vi "Local Bus Termination.vi"(8 "error in (no error)":errorcluster, 11 "BoardHandle":T1) -> (0 "error out":errorcluster, 2 "Local Bus Termination ON?":bool, 3 "BoardHandle out":T1)   [LabVIEW 2020, in "CAEN PSM.lvlib"]
doc: "This function returns bus termination status. (This is supported by NIM / DESKTOP HV family)."
uses:
  CAEN PSM.lvlib
  Private/BoardHandle.ctl
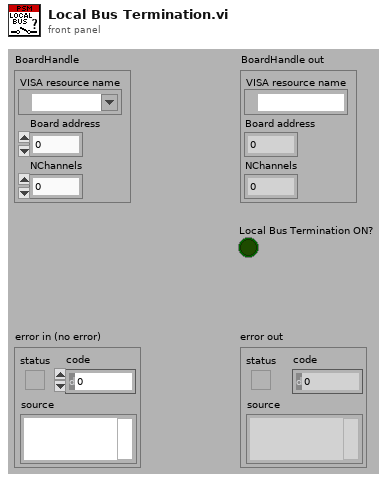
[diagram p1: front panel]
types:
  T1 = typedef "CAEN PSM.lvlib/BoardHandle.ctl" = cluster{"VISA resource name":refnum<visa-resource-name>, "Board address":i8, "NChannels":u8}
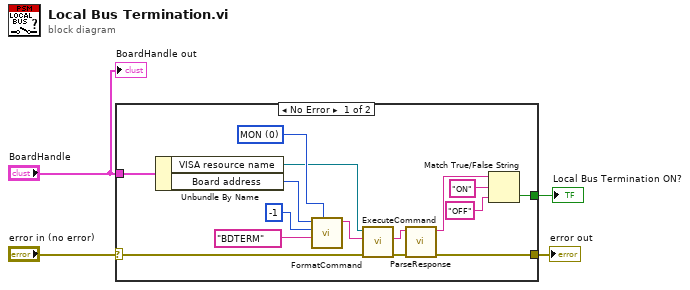
[diagram p0: block diagram]
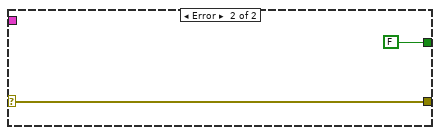
[diagram p2: hidden frame]
diagram:
  n1 = case shown="No Error" "error in (no error)" {
    selector: "error in (no error)" -> [w11 w21]
    tunnel: [w14 w21] -> w3
    tunnel: "BoardHandle" -> [w12 _]
    tunnel: [w5 FALSE ("selection")] -> w1
    frame No Error {
      w18 = u8 0 items=["MON", "SET"] ("CMD")
      n2 = Unbundle By Name(w12) -> ("VISA resource name"=w17:refnum<visa-resource-name>, "Board address"=w19:i8)
      n3 = call "FormatCommand.vi"("CMD (MON)"=w18, "PAR"="BDTERM", "CH"=i8 -1, "BD (0)"=w19) -> ("cmd"=w16:string)  [unwired: 7 in]
      n4 = call "ExecuteCommand.vi"("error in (no error)"=w11, "Command"=w16, "VISA resource name"=w17) -> ("error out"=w15:errorcluster, "Response"=w13:string)  [unwired: 6 in, 1 out]
      n5 = call "ParseResponse.vi"("error in (no error)"=w15, "Response"=w13) -> ("error out"=w14:errorcluster, "val"=w8:string)  [unwired: 6 in, 2 out]
      n6 = Match True/False String(2:"OFF" ("false string"), 3:"ON" ("true string"), 4:w8) -> (0:w5:bool)  [unwired: 1 out]
    }
    frame Error {
    }
  }
  "error out" <- w3
  "Local Bus Termination ON?" <- w1
  "BoardHandle out" <- "BoardHandle"
